vi "PowerStatusChanged.vi"(7 "ControlQueue":refnum<queue>, 8 "error in (no error)":errorcluster, 9 "PowerStatus":bool, 10 "PowerStatusChanged":bool, 11 "DAQmxTaksContainer_General in":refnum<class "DAQmxTaksContainer_General.lvclass">) -> (0 "error out":errorcluster, 3 "DAQmxTaksContainer_General out":refnum<class "DAQmxTaksContainer_General.lvclass">)   [LabVIEW 2015, in "DAQmxTaksContainer_General.lvclass"]
uses:
  DAQmxTaksContainer_General.lvclass
  dependecies/ControlsVIs/Clusters-def/ProtypeCommand-DAQmxReply.ctl
  dependecies/ControlsVIs/Clusters-def/SERVER-Commands.ctl
  dependecies/ControlsVIs/Clusters-def/Standard Command.ctl
  DAQmxTaksContainer_General.lvclass/DAQmxTaksContainer_General.ctl
  Control/Control-Server/Control-Server.lvclass
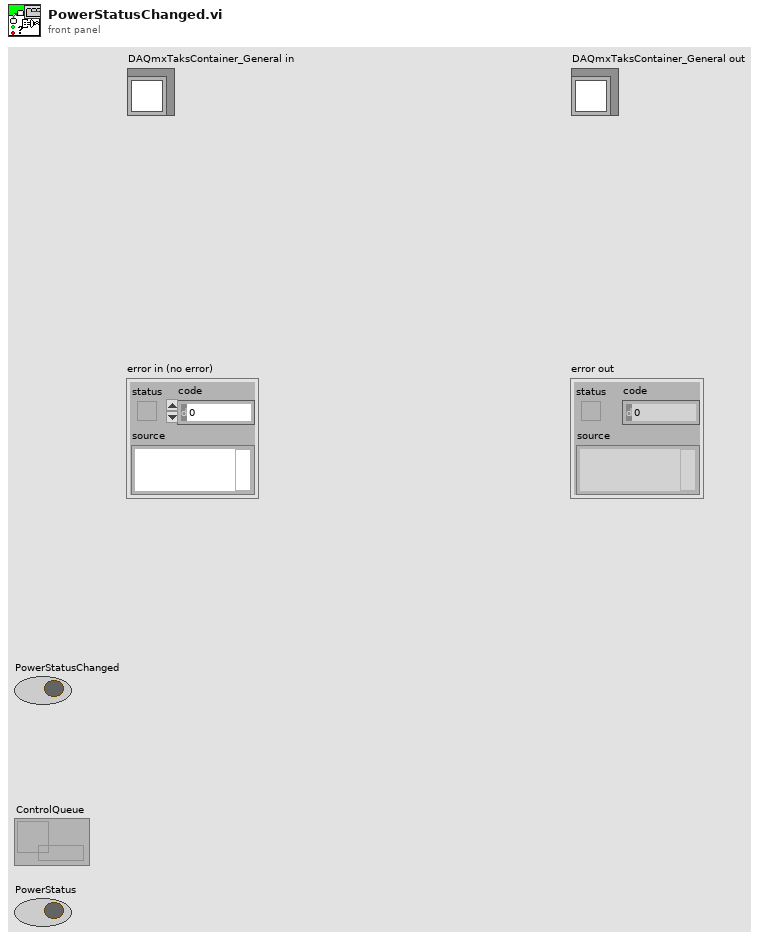
[diagram p1: front panel]
types:
  T1 = typedef "Standard Command.ctl" = cluster{"command":string, "data":variant}
  T2 = typedef "Control-Server.lvclass/SERVER-Commands.ctl" = string
  T3 = typedef "ProtypeCommand-DAQmxReply.ctl" = cluster{"On/Off":bool, "error out":errorcluster}
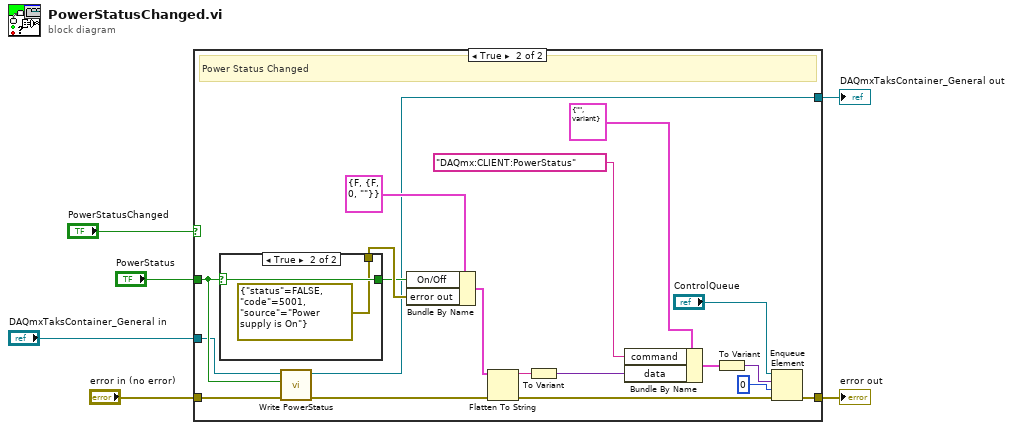
[diagram p0: block diagram]
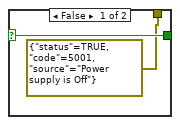
[diagram p3: hidden frame]
diagram:
  n1 = case shown="True" "PowerStatusChanged" {
    tunnel: "DAQmxTaksContainer_General in" -> [w8 w11]
    tunnel: [w8 w12] -> w4
    tunnel: "error in (no error)" -> [w7 w10]
    tunnel: [w7 w19] -> w3
    tunnel: "PowerStatus" -> [_ w13]
    frame False {
    }
    frame True {
      # "Power Status Changed"
      n2 = case shown="True" w13 {
        selector: w13 -> [w29 w31]
        tunnel: [w29 w31] -> w21
        tunnel: [errorcluster {"status"=TRUE, "code"=5001, "source"="Power supply is Off"} ("error out") errorcluster {"status"=FALSE, "code"=5001, "source"="Power supply is On"} ("error out")] -> w22
        frame False {
        }
        frame True {
        }
      }
      n3 = call "Write PowerStatus.vi"("error in (no error)"=w10, "PowerStatus"=w13, "DAQmxTaksContainer_General in"=w11) -> ("error out"=w9:errorcluster, "DAQmxTaksContainer_General out"=w12:refnum<class "DAQmxTaksContainer_General.lvclass">)  [unwired: 7 in]
      n4 = Bundle By Name(cluster=T3 {"On/Off"=FALSE, "error out"={"status"=FALSE, "code"=0, "source"=""}} ("output cluster"), "On/Off"=w21, "error out"=w22) -> (w26:T3)
      n5 = Flatten To String(anything=w26, error in (no error)=w9) -> (data string=w24:string, error out=w20:errorcluster)  [unwired: 2 in, 1 out]
      n6 = To Variant(anything=w24) -> (Variant=w25:variant)
      n7 = Bundle By Name(cluster=T1 {"command"="", "data"=variant} ("input cluster"), "command"=T2 "DAQmx:CLIENT:PowerStatus" ("Commands"), "data"=w25) -> (w18:T1)
      n8 = To Variant(anything=w18) -> (Variant=w17:variant)
      n9 = Enqueue Element(queue="ControlQueue", element=w17, timeout in ms (-1)=0 ("timeout en ms (-1)"), error in (no error)=w20) -> (error out=w19:errorcluster)  [unwired: 2 out]
    }
  }
  "error out" <- w3
  "DAQmxTaksContainer_General out" <- w4
